vi "Untitled 1.vi"() -> ()   [LabVIEW 2021]
panel:
  in  "Stop Button":bool
  out "Variable1":string
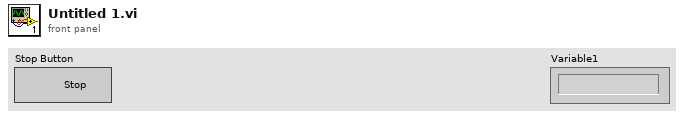
[diagram p1: front panel]
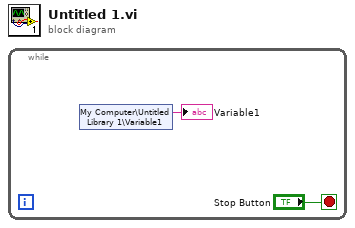
[diagram p0: block diagram]
diagram:
  n1 = while {
    stop <- "Stop Button" stop-if-true
    n2 = shared-variable "My Computer\\Untitled Library 1\\Variable1"() -> (→"Variable1":string)  [unwired: 1 in, 1 out]
  }
